vi "03T_inputPacketParsing.vi"(11 "string":string) -> (0 "TrigTimer, s":dbl, 1 "Service":cluster{i32, i32, i32, i32}, 2 "Voltage":cluster{dbl, dbl}, 3 "Temp":cluster{dbl, dbl, dbl})   [LabVIEW 2013]
panel:
  out "Temp, K":dbl
  out "Temp_sp, K":dbl
  out "Temp_gsp, K":dbl
  out "Vout, V":dbl
  out "Vin, V":dbl
  out "serv1":i32
  out "serv2":i32
  out "serv3":i32
  out "serv4":i32
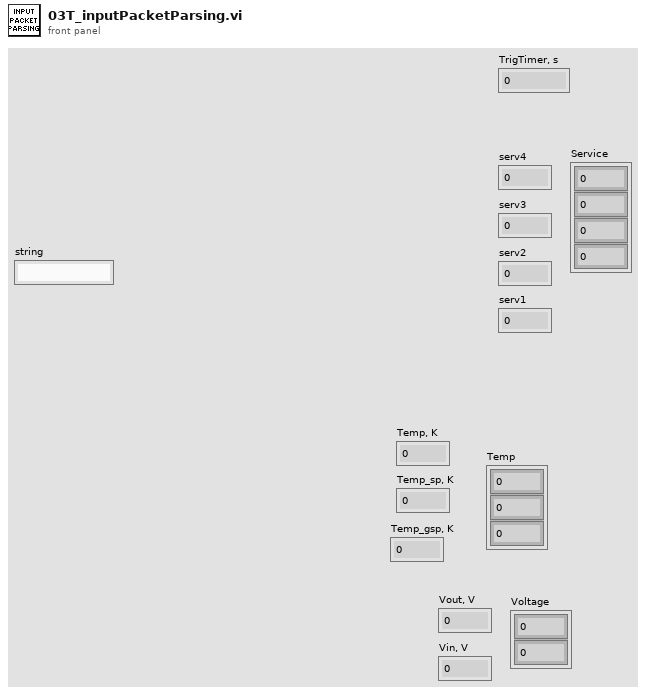
[diagram p1: front panel]
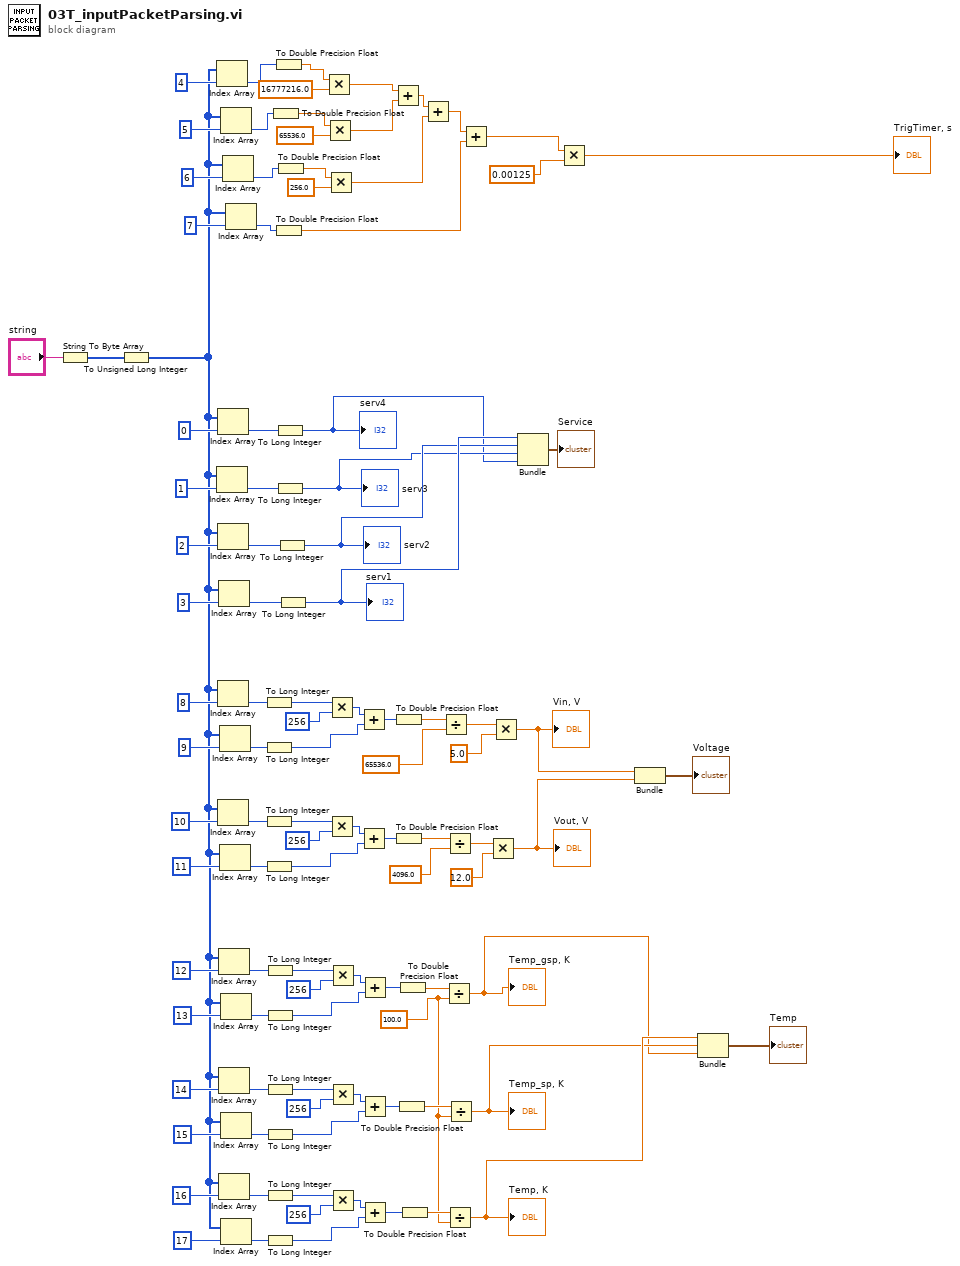
[diagram p0: block diagram]
diagram:
  w18 = 100.0 ("y")
  n1 = String To Byte Array(string="string") -> (unsigned byte array=w74:u8[])
  n2 = To Unsigned Long Integer(number=w74) -> (unsigned 32bit integer=w25:u32[])
  n3 = Index Array(array=w25, index=4) -> (element=w80:u32)
  n4 = Index Array(array=w25, index=1) -> (element=w69:u32)
  n5 = Index Array(array=w25, index=0) -> (element=w72:u32)
  n6 = Index Array(array=w25, index=2) -> (element=w70:u32)
  n7 = Index Array(array=w25, index=8) -> (element=w67:u32)
  n8 = Index Array(array=w25, index=10) -> (element=w54:u32)
  n9 = Index Array(array=w25, index=3) -> (element=w71:u32)
  n10 = Index Array(array=w25, index=12) -> (element=w46:u32)
  n11 = Index Array(array=w25, index=14) -> (element=w38:u32)
  n12 = Index Array(array=w25, index=16) -> (element=w30:u32)
  n13 = Index Array(array=w25, index=9) -> (element=w68:u32)
  n14 = Index Array(array=w25, index=11) -> (element=w55:u32)
  n15 = Index Array(array=w25, index=5) -> (element=w81:u32)
  n16 = Index Array(array=w25, index=13) -> (element=w47:u32)
  n17 = Index Array(array=w25, index=15) -> (element=w39:u32)
  n18 = Index Array(array=w25, index=17) -> (element=w31:u32)
  n19 = Index Array(array=w25, index=6) -> (element=w84:u32)
  n20 = Index Array(array=w25, index=7) -> (element=w86:u32)
  n21 = To Long Integer(number=w67) -> (32bit integer=w66:i32)
  n22 = To Long Integer(number=w68) -> (32bit integer=w63:i32)
  n23 = To Long Integer(number=w54) -> (32bit integer=w53:i32)
  n24 = To Long Integer(number=w55) -> (32bit integer=w50:i32)
  n25 = To Long Integer(number=w46) -> (32bit integer=w45:i32)
  n26 = To Long Integer(number=w47) -> (32bit integer=w42:i32)
  n27 = To Long Integer(number=w38) -> (32bit integer=w37:i32)
  n28 = To Long Integer(number=w39) -> (32bit integer=w34:i32)
  n29 = To Long Integer(number=w30) -> (32bit integer=w29:i32)
  n30 = To Long Integer(number=w31) -> (32bit integer=w26:i32)
  n31 = To Double Precision Float(number=w81) -> (double precision float=w82:dbl)
  n32 = To Double Precision Float(number=w80) -> (double precision float=w79:dbl)
  n33 = To Double Precision Float(number=w86) -> (double precision float=w85:dbl)
  n34 = To Long Integer(number=w72) -> (32bit integer=w59:i32)
  "serv4" <- w59
  n35 = To Long Integer(number=w69) -> (32bit integer=w60:i32)
  "serv3" <- w60
  n36 = To Double Precision Float(number=w84) -> (double precision float=w83:dbl)
  n37 = To Long Integer(number=w70) -> (32bit integer=w61:i32)
  "serv2" <- w61
  n38 = To Long Integer(number=w71) -> (32bit integer=w62:i32)
  "serv1" <- w62
  n39 = Multiply(x=w79, y=16777216.0) -> (x*y=w94:dbl)
  n40 = Multiply(x=w82, y=65536.0) -> (x*y=w93:dbl)
  n41 = Multiply(x=w83, y=256.0) -> (x*y=w91:dbl)
  n42 = Multiply(x=w66, y=256) -> (x*y=w64:i32)
  n43 = Multiply(x=w53, y=256) -> (x*y=w51:i32)
  n44 = Multiply(x=w45, y=256) -> (x*y=w43:i32)
  n45 = Multiply(x=w37, y=256) -> (x*y=w35:i32)
  n46 = Multiply(x=w29, y=256) -> (x*y=w27:i32)
  n47 = Add(x=w64, y=w63) -> (x+y=w12:i32)
  n48 = Add(x=w51, y=w50) -> (x+y=w13:i32)
  n49 = Add(x=w43, y=w42) -> (x+y=w24:i32)
  n50 = Add(x=w35, y=w34) -> (x+y=w23:i32)
  n51 = Add(x=w27, y=w26) -> (x+y=w22:i32)
  n52 = Add(x=w94, y=w93) -> (x+y=w92:dbl)
  n53 = To Double Precision Float(number=w12) -> (double precision float=w11:dbl)
  n54 = To Double Precision Float(number=w13) -> (double precision float=w9:dbl)
  n55 = To Double Precision Float(number=w23) -> (double precision float=w20:dbl)
  n56 = To Double Precision Float(number=w24) -> (double precision float=w21:dbl)
  n57 = To Double Precision Float(number=w22) -> (double precision float=w19:dbl)
  n58 = Add(x=w92, y=w91) -> (x+y=w90:dbl)
  n59 = Divide(x=w11, y=65536.0) -> (x/y=w10:dbl)
  n60 = Divide(x=w21, y=w18) -> (x/y=w15:dbl)
  "Temp_gsp, K" <- w15
  n61 = Divide(x=w9, y=4096.0) -> (x/y=w6:dbl)
  n62 = Divide(x=w19, y=w18) -> (x/y=w17:dbl)
  "Temp, K" <- w17
  n63 = Divide(x=w20, y=w18) -> (x/y=w16:dbl)
  "Temp_sp, K" <- w16
  n64 = Add(x=w90, y=w85) -> (x+y=w77:dbl)
  n65 = Multiply(x=w6, y=12.0) -> (x*y=w2:dbl)
  "Vout, V" <- w2
  n66 = Multiply(x=w10, y=5.0) -> (x*y=w3:dbl)
  "Vin, V" <- w3
  n67 = Bundle(w62, w61, w60, w59) -> (→"Service":cluster{i32, i32, i32, i32})  [unwired: 1 in]
  n68 = Multiply(x=w77, y=0.00125) -> (x*y=→"TrigTimer, s":dbl)
  n69 = Bundle(w3, w2) -> (→"Voltage":cluster{dbl, dbl})  [unwired: 1 in]
  n70 = Bundle(w17, w16, w15) -> (→"Temp":cluster{dbl, dbl, dbl})  [unwired: 1 in]
